vi "GetVisibillitySettings.vi"(0 "reference":refnum<class "ClassNode.lvclass">, 5 "error in (no error)":errorcluster) -> (14 "reference out":refnum<class "ClassNode.lvclass">, 15 "showAttribute":bool, 16 "showMethods":bool, 19 "error out":errorcluster)   [LabVIEW 2012, in "ClassNode.lvclass"]
doc: "GetVisibillitySettings"
uses:
  <resource>/Framework/Providers/Open_GDS/UML/ClassNode_class/ClassNode.lvclass
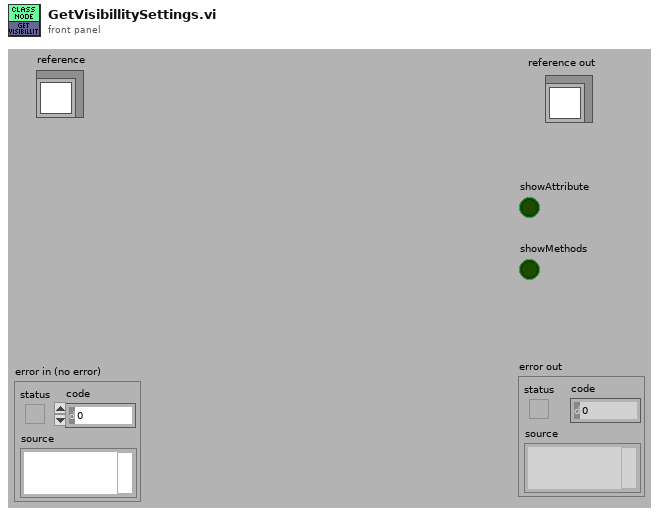
[diagram p1: front panel]
types:
  T1 = typedef "ClassNode.lvclass/ObjectAttributes.ctl" = cluster{"Base class":T2, "midHeight":dbl, "botHeight":dbl, "name":refnum<class "MultiLineString.lvclass">, "attributes":refnum<class "MultiLineString.lvclass">, "methods":refnum<class "MultiLineString.lvclass">, "DEFAULT_COMPARTMENT_HEIGHT":i32, "DEFAULT_WIDTH":i32, "DEFAULT_HEIGHT":i32, "showMethods":bool, "showAttributes":bool, "ClassPath":path}
  T2 = typedef "RectangularNode.lvclass/ObjectAttributes.ctl" = cluster{"Base class":T3, "bounds":T4}
  T3 = typedef "AbstractNode.lvclass/ObjectAttributes.ctl" = cluster{"parent":refnum<class "AbstractNode.lvclass">, "children":refnum<class "AbstractNode.lvclass">[], "Hidden":bool}
  T4 = typedef "Rectangle Rectangle2D.ctl" = cluster{"x":dbl, "y":dbl, "width":dbl, "height":dbl}
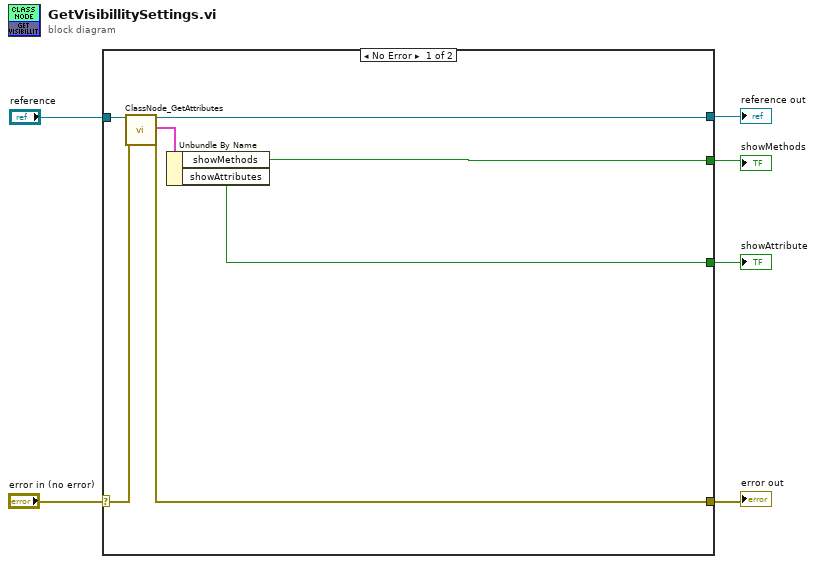
[diagram p0: block diagram]
diagram:
  n1 = case shown="No Error" "error in (no error)" {
    selector: "error in (no error)" -> [w13 w14]
    tunnel: "reference" -> [w12 w15]
    tunnel: [w9 w14] -> w4
    tunnel: [w10 w15] -> w3
    tunnel: [w8 _] -> w2
    tunnel: [w7 _] -> w1
    frame No Error {
      n2 = call <resource>:"ClassNode_GetAttributes.vi"("reference in"=w12, "error in (no error)"=w13) -> ("reference out"=w10:refnum<class "ClassNode.lvclass">, "Attributes"=w11:T1, "error out"=w9:errorcluster)  [unwired: 15 out]
      n3 = Unbundle By Name(w11) -> ("showMethods"=w8:bool, "showAttributes"=w7:bool)
    }
    frame Error {
    }
  }
  "reference out" <- w3
  "error out" <- w4
  "showMethods" <- w2
  "showAttribute" <- w1
